vi "begin direct read.vi"(5 "id":u32, 7 "event":refnum<user-event>, 8 "error in":errorcluster, 9 "bytes to read":u32, 11 "socket":u64) -> (0 "error out":errorcluster)   [LabVIEW 2016, in "async tls dl.lvlib"]
uses:
  async tls dl.lvlib
  tls data user event.ctl
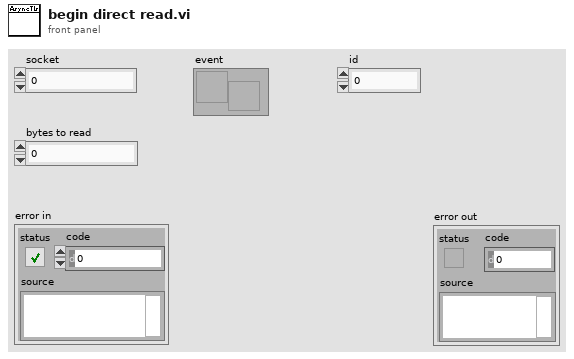
[diagram p1: front panel]
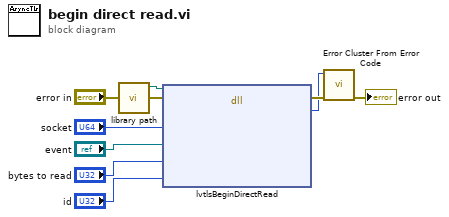
[diagram p0: block diagram]
diagram:
  n1 = call "library path.vi"() -> ("path"=w1:path)  [unwired: 11 in]
  n2 = dll-call lib="C:/Users/IEUser/Desktop/libasynclvtls/lvasynctls.dll" fn="lvtlsBeginDirectRead"(path in=w1, error in="error in", "socket"="socket", "event"="event", "bytes to read"="bytes to read", "id"="id") -> (error out=w9:errorcluster, "err"=w8:i32)  [unwired: 5 in, 1 out]
  n3 = call <vilib>:"Error Cluster From Error Code.vi"("error in (no error)"=w9, "error code (0)"=w8) -> ("error out"=→"error out":errorcluster)  [unwired: 7 in]
